vi "Close.vi"(8 "error in (no error)":errorcluster, 11 "SLSC Switch in":refnum<class "SLSC Switch.lvclass">) -> (0 "error out":errorcluster)   [LabVIEW 2016, in "SLSC Switch.lvlib" / "SLSC Switch.lvclass"]
doc: "Disconnects all channels and terminates the SLSC-SWITCH session and all of its attributes and deallocates any memory resources the driver uses."
uses:
  SLSC Switch.lvclass
  SLSC Switch.lvclass/SLSC Switch.ctl
  <vilib>/National Instruments/SLSC Local or Remote Interface/SLSC Interface Class/SLSC Interface.lvclass
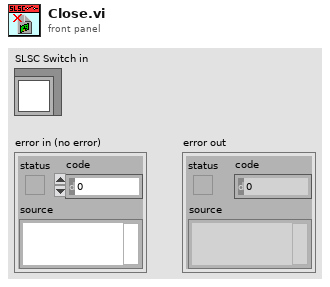
[diagram p1: front panel]
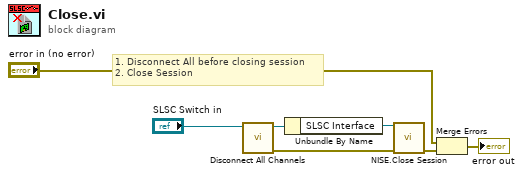
[diagram p0: block diagram]
diagram:
  # "1. Disconnect All before closing session\n2. Close Session"
  n1 = call "Disconnect All Channels.vi"("SLSC Switch in"="SLSC Switch in") -> ("error out"=w4:errorcluster, "SLSC Switch out"=w6:refnum<class "SLSC Switch.lvclass">)  [unwired: 9 in]
  n2 = Unbundle By Name(w6) -> ("SLSC Interface"=w5:refnum<class "SLSC Interface.lvclass">)
  n3 = call <vilib>:"NISE.Close Session.vi"("SLSC Interface in"=w5, "error in (no error)"=w4) -> ("error out"=w2:errorcluster)  [unwired: 13 in]
  n4 = Merge Errors("error in (no error)", w2) -> (→"error out":errorcluster)
